vi "ClawNetwork.vi"(8 "error in (no error)":errorcluster) -> (0 "error out":errorcluster)   [LabVIEW 2020]
doc: "Claw network\n\nInputs:\n -- Error in -- Error cluster -- propagated error input\n\nOutputs:\n -- Error out -- Error cluster -- progated error output"
uses:
  ClawGlobal.vi
  <vilib>/Rock Robotics/Network Tables/NT Write Boolean.vi
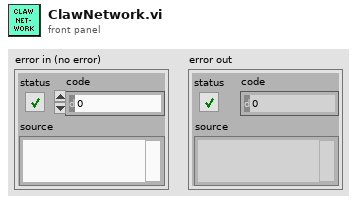
[diagram p1: front panel]
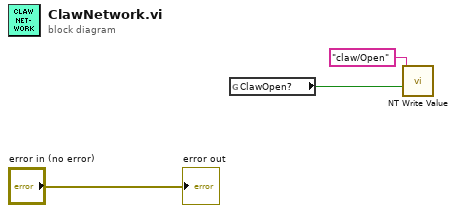
[diagram p0: block diagram]
diagram:
  n1 = global read "ClawGlobal.vi" "ClawOpen?"() -> (w2:bool)
  n2 = call-poly <vilib>:"NT Write Value.vi"("value"=w2, "name"="claw/Open") -> ()  [unwired: 9 in, 1 out]
  "error out" <- "error in (no error)"
